vi "Find image index.vi"(8 "error in (no error)":errorcluster, 9 "ID":u8, 11 "Save Image in":refnum<class "Save Image.lvclass">) -> (0 "error out":errorcluster, 3 "Save Image in":refnum<class "Save Image.lvclass">)   [LabVIEW 2018, in "Save Image.lvclass"]
uses:
  Save Image.lvclass
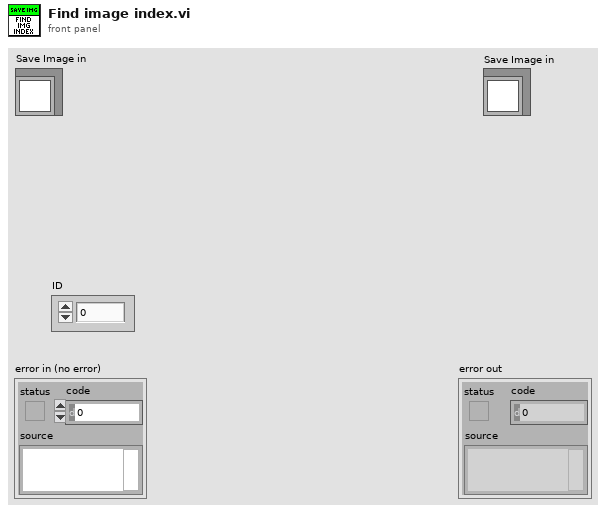
[diagram p1: front panel]
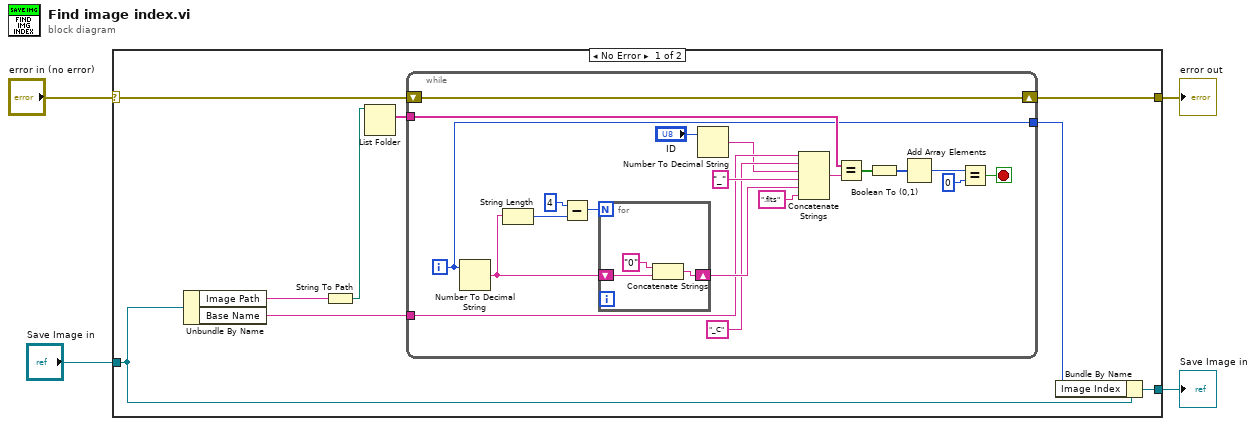
[diagram p0: block diagram]
diagram:
  n1 = case shown="No Error" "error in (no error)" {
    selector: "error in (no error)" -> [w8 w38]
    tunnel: [w10 w38] -> w3
    tunnel: [w9 w37] -> w1
    tunnel: "Save Image in" -> [w7 w37]
    frame No Error {
      n2 = Unbundle By Name(w7) -> ("Image Path"=w6:string, "Base Name"=w5:string)
      n3 = String To Path(string=w6) -> (path=w13:path)
      n4 = List Folder(path=w13) -> (filenames=w12:string[])  [unwired: 3 in, 3 out]
      n5 = while {
        tunnel: w12 -> [w21]
        shift-right: [w20] -> w10
        shift-left: w8 -> [w20]
        tunnel: [w18] -> w11
        tunnel: w5 -> [w17]
        i -> [w18]
        stop <- w29 stop-if-true
        n6 = Number To Decimal String(number=w18) -> (decimal integer string=w22:string)  [unwired: 1 in]
        n7 = String Length(string=w22) -> (length=w25:i32)
        n8 = Subtract(x=4, y=w25) -> (x-y=w26:i32)
        n9 = for {
          N: w26 -> [_]
          shift-right: [w36] -> w23
          shift-left: w22 -> [w34]
          n10 = Concatenate Strings("0" ("string"), w34) -> (w36:string)
        }
        n11 = Number To Decimal String(number="ID") -> (decimal integer string=w14:string)  [unwired: 1 in]
        n12 = Concatenate Strings(w17, "_C", w14, "_" ("string"), w23, ".fits" ("string")) -> (w19:string)
        n13 = Equal?(x=w21, y=w19) -> (x = y?=w33:bool[])
        n14 = Boolean To (0,1)(Boolean=w33) -> (0, 1=w32:i16[])
        n15 = Add Array Elements(numeric array=w32) -> (sum=w31:i16)
        n16 = Equal?(x=w31, y=0) -> (x = y?=w29:bool)
      }
      n17 = Bundle By Name(cluster=w7, "Image Index"=w11) -> (w9:refnum<class "Save Image.lvclass">)
    }
    frame Error {
    }
  }
  "error out" <- w3
  "Save Image in" <- w1
